vi "Move Robot.vi"   [LabVIEW 2016, in "Moving Motor.lvrbt"]
uses:
  Moving Motor.lvrbt
  <vilib>/NXT/Hardware/Plugins/Tetrix DC Motor/TetrixDCMotorAddress.ctl
  <vilib>/NXT/NXTIO Xnodes/NXTIONodeSubVIs/TETRIX IO Move DC Motors.vi
  <vilib>/NXT/NXTIO Xnodes/NXTIONodeSubVIs/LEGOStopAllMotors.vi
  <vilib>/NXT/Subs/LVHSConnector.ctl
  <vilib>/NXT/NXTIO Xnodes/AddressXNode/NXTIOAddress.xnode
  <vilib>/NXT/NXTIO Xnodes/NXTIOXNode/NXTIO.xnode
  <vilib>/NXT/Hardware/Plugins/Tetrix 180 deg Servo/Tetrix180ServoAddress.ctl
  <vilib>/NXT/LegoClasses/BrickReference/BrickReference.lvclass
types:
  T1 = typedef "TetrixDCMotorAddress.ctl" = i32
  T2 = typedef "LVHSConnector.ctl" = refnum<class "BrickReference.lvclass">
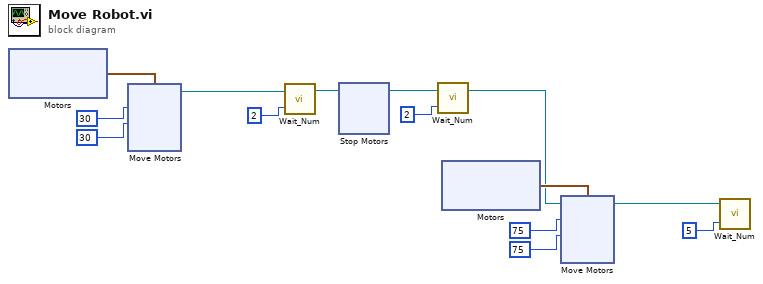
[diagram p0: block diagram]
diagram:
  n1 = xnode "Motors"() -> ("Motor"=w14:cluster{"TetrixDCMotor":T1, "TetrixDCMotor":T1})
  n2 = xnode "Move Motors"("Power/Speed 2"=30, "Power/Speed 1"=30, "Motors"=w14) -> ("NXT/EV3"=w11:T2)  [unwired: 1 in]
  n3 = call <vilib>:"Wait_Num.vi"("Time (1 sec)"=2, "NXT/EV3"=w11) -> ("NXT/EV3"=w4:T2)  [unwired: 2 in]
  n4 = xnode "Stop Motors"("NXT/EV3"=w4) -> ("NXT/EV3"=w2:T2)  [unwired: 1 in]
  n5 = call <vilib>:"Wait_Num.vi"("Time (1 sec)"=2, "NXT/EV3"=w2) -> ("NXT/EV3"=w1:T2)  [unwired: 2 in]
  n6 = xnode "Motors"() -> ("Motor"=w9:cluster{"TetrixDCMotor":T1, "TetrixDCMotor":T1})
  n7 = xnode "Move Motors"("Power/Speed 2"=75, "Power/Speed 1"=75, "Motors"=w9, "NXT/EV3"=w1) -> ("NXT/EV3"=w5:T2)
  n8 = call <vilib>:"Wait_Num.vi"("Time (1 sec)"=5, "NXT/EV3"=w5) -> ()  [unwired: 2 in, 1 out]
